vi "niScope Read Measurement.vi"(0 "instrument handle":refnum<k15>, 1 "timeout":dbl=5.0 format="%.2f", 5 "channels":string="0", 7 "scalar measurement":T1=4000 items=["None"=4000, "Frequency"=2, "Average Frequency"=1016, "FFT Frequency"=1008, "Period"=3, "Average Period"=1015, "Rise Time"=0, "Fall Time"=1, "Rising Slew Rate"=1010, "Falling Slew Rate"=1011, "Overshoot"=18, "Preshoot"=19, "Voltage RMS"=4, "Voltage Cycle RMS"=16, "AC Estimate"=1012, "FFT Amplitude"=1009, "Voltage Average"=10, "Voltage Cycle Average"=17, "DC Estimate"=1013, "Voltage Max"=6, "Voltage Min"=7, "Voltage Peak-to-Peak"=5, "Voltage High"=8, "Voltage Low"=9, "Voltage Amplitude"=15, "Voltage Top"=1007, "Voltage Base"=1006, "Voltage Base-to-Top"=1017, "Negative Width"=11, "Positive Width"=12, "Negative Duty Cycle"=13, "Positive Duty Cycle"=14, "Integral"=1005, "Area"=1003, "Cycle Area"=1004, "Time Delay"=1014, "Phase Delay"=1018, "Low Ref Volts"=1000, "Mid Ref Volts"=1001, "High Ref Volts"=1002, "Volt. Hist. Mean"=2000, "Volt. Hist. Stdev"=2001, "Volt. Hist. Median"=2003, "Volt. Hist. Mode"=2010, "Volt. Hist. Max"=2005, "Volt. Hist. Min"=2006, "Volt. Hist. Peak-to-Peak"=2002, "Volt. Hist. Mean + Stdev"=2007, "Volt. Hist. Mean + 2 Stdev"=2008, "Volt. Hist. Mean + 3 Stdev"=2009, "Volt. Hist. Hits"=2004, "Volt. Hist. New Hits"=2011, "Time Hist. Mean"=3000, "Time Hist. Stdev"=3001, "Time Hist. Median"=3003, "Time Hist. Mode"=3010, "Time Hist. Max"=3005, "Time Hist. Min"=3006, "Time Hist. Peak-to-Peak"=3002, "Time Hist. Mean + Stdev"=3007, "Time Hist. Mean + 2 Stdev"=3008, "Time Hist. Mean + 3 Stdev"=3009, "Time Hist. Hits"=3004, "Time Hist. New Hits"=3011], 11 "error in":errorcluster) -> (4 "instrument handle out":refnum<k15>, 6 "result":dbl format="%.2f", 15 "error out":errorcluster)   [LabVIEW 2011]
doc: "Initiates an acquisition, waits for it to complete, and performs the specified waveform measurement for a single channel and record."
uses:
  <instrlib>/niScope/Controls/niScope scalar measurement.ctl
  niScope_32.dll
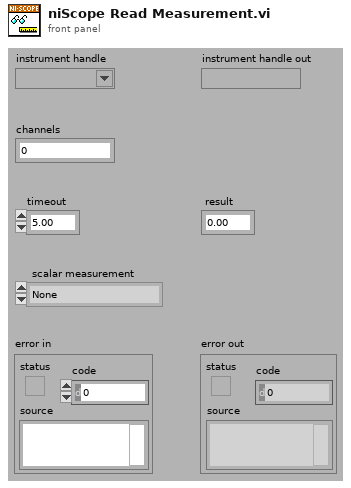
[diagram p1: front panel]
types:
  T1 = typedef "niScope scalar measurement.ctl" = i32
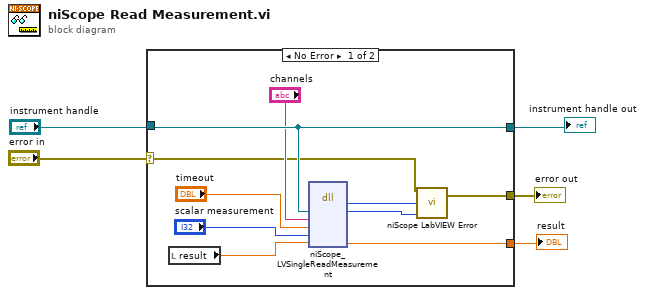
[diagram p0: block diagram]
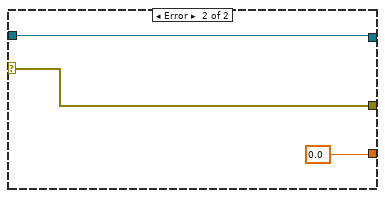
[diagram p2: hidden frame]
diagram:
  n1 = case shown="No Error" "error in" {
    selector: "error in" -> [w6 w16]
    tunnel: [w15 w16] -> w5
    tunnel: [w11 0.0] -> w2
    tunnel: "instrument handle" -> [w12 w18]
    tunnel: [w12 w18] -> w4
    frame No Error {
      n2 = local read "result"() -> (w7:dbl)
      n3 = dll-call lib="niScope_*.*" fn="niScope_LVSingleReadMeasurement"("instrument handle"=w12, "channel"="channels", "timeout"="timeout", "scalarMeasFunction"="scalar measurement", "result"=w7) -> ("status"=w14:i32, "instrument handle"=w13:u32, "result"=w11:dbl)  [unwired: 6 in, 2 out]
      n4 = call <instrlib>:"niScope LabVIEW Error.vi"("instrument handle"=w13, "niScope error code (0)"=w14, "error in (no error)"=w6) -> ("error out"=w15:errorcluster)  [unwired: 2 in]
    }
    frame Error {
    }
  }
  "instrument handle out" <- w4
  "error out" <- w5
  "result" <- w2
